vi "get_device_info_base.vi"(7 "info_options":T1, 9 "device_index":i32, 11 "error in (no error)":errorcluster, 12 "dialog? (T)":bool=TRUE) -> (8 "retrieved_info (str)":string, 15 "error out":errorcluster)   [LabVIEW 2020, in "classes.lvlib" / "_Controller.lvclass"]
doc: "Retrieves device info based on device index. Device index is directly related to the order of all items found. \n\nImplementss the USB Communication API function \"fnPerformaxComGetProductString\".\n\nProduced By:\n\nChristopher Lemieux\nKod Integrations, LLC\n4835 Marianne Drive\nMount Airy, MD 21771\nhttp://www.kodintegrations.com\nemail: clemieux@kodintegrations.com\nphone: (240) 687-1288"
uses:
  _Controller.lvclass
  device_info_options.ctl
  translate_to_from_byte_array_actions.ctl
  error_actions.ctl
  PerformaxCom.dll
  common.lvlib
panel:
  in  "initialized_array":u8[](array[numeric])
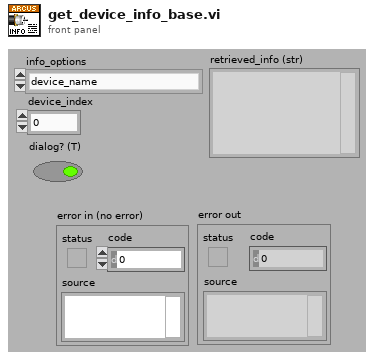
[diagram p1: front panel]
types:
  T1 = typedef "common.lvlib/device_info_options.ctl" = enum16{"device_name", "description"}
  T2 = typedef "common.lvlib/translate_to_from_byte_array_actions.ctl" = enum16{"to_bytes", "to_string"}
  T3 = typedef "common.lvlib/error_actions.ctl" = enum16{"clearBuff", "closeRef", "nodeErr", "noDeviceInfo", "noDevices", "openRef", "sendReceive", "setTimeouts", "unknown"}
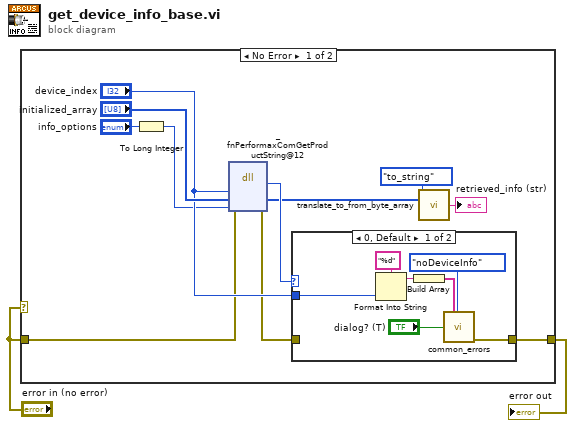
[diagram p0: block diagram]
diagram:
  n1 = case shown="No Error" "error in (no error)" {
    tunnel: "error in (no error)" -> [w4 w22]
    tunnel: [w11 w22] -> w1
    frame No Error {
      n2 = To Long Integer(number="info_options") -> (32bit integer=w5:i32)
      n3 = dll-call lib="PerformaxCom.dll" fn="_fnPerformaxComGetProductString@12"(error in=w4, "devInd"="device_index", "returnedInfo"="initialized_array", "options"=w5) -> (error out=w3:errorcluster, w12:i32, "returnedInfo"=w9:u8[])  [unwired: 4 in, 1 out]
      n4 = case shown="0, Default" w12 {
        tunnel: [w19 w21] -> w11
        tunnel: w3 -> [_ w21]
        tunnel: "device_index" -> [w18 _]
        frame 0, Default {
          n5 = Format Into String(format string="%d", w18) -> (resulting string=w16:string)  [unwired: 2 in, 1 out]
          n6 = Build Array(w16) -> (w15:string[])
          n7 = call "common_errors.vi"("common_errors"=error_actions."noDeviceInfo" ("errors"), "dialog? (T)"="dialog? (T)", "supp_text"=w15) -> ("error out"=w19:errorcluster)  [unwired: 12 in]
        }
        frame 1 {
        }
      }
      n8 = call "translate_to_from_byte_array.vi"("actions"=translate_to_from_byte_array_actions."to_string", "byte_array (in)"=w9) -> ("string (out)"=→"retrieved_info (str)":string)  [unwired: 12 in, 1 out]
    }
    frame Error {
    }
  }
  "error out" <- w1
